vi "save default config.vi"() -> (3 "Data out":T1)   [LabVIEW 2025]
uses:
  safety light settings.ctl
  8253c311-8266-41c7-aa3e-9534f31a7151.vi
  fc13ce0c-d746-4782-a37b-4bbc89a20136.vi
  <vilib>/JDP Science/JSONtext/Variant to JSON Text.vi
  <vilib>/JDP Science/JSONtext/JSON text to Variant.vi
  <vilib>/JDP Science/JSONtext/LVClass Serializer/JSONtext LVClass Serializer.lvclass
panel:
  in  "overwrite file":bool
  in  "default config":T1
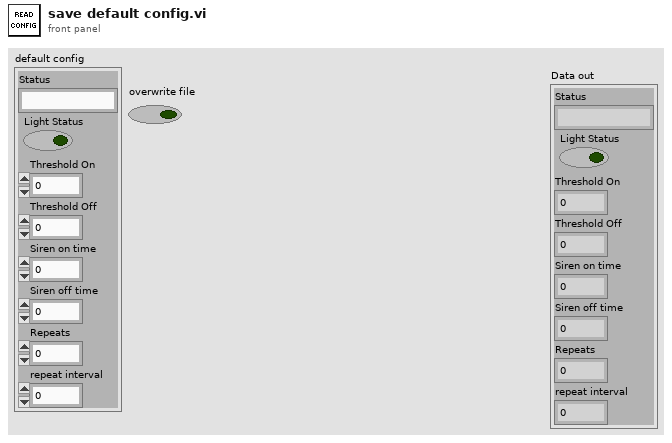
[diagram p1: front panel]
types:
  T1 = typedef "safety light settings.ctl" = cluster{"Status":string, "Light Status":bool, "Threshold On":dbl, "Threshold Off":dbl, "Siren on time":dbl, "Siren off time":dbl, "Repeats":i32, "repeat interval":dbl}
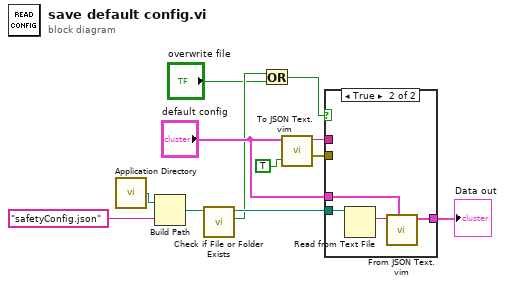
[diagram p0: block diagram]
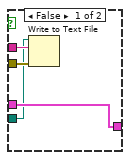
[diagram p2: hidden frame]
diagram:
  n1 = call <vilib>:"Application Directory.vi"() -> ("Application Directory"=w12:path)
  n2 = Build Path(base path=w12, name or relative path="safetyConfig.json" ("JSON string")) -> (appended path=w10:path)
  n3 = call <vilib>:"Check if File or Folder Exists.vi"("path"=w10) -> ("file or folder exists?"=w4:bool, "dup path"=w9:path)  [unwired: 8 in, 1 out]
  n4 = Or(x=w4, y="overwrite file") -> (x .or. y?=w2:bool)
  n5 = call "To JSON Text.vim"("Pretty Print?"=TRUE, "Anything"="default config") -> ("error out"=w6:errorcluster, "<JSON>"=w7:string)  [unwired: 8 in]
  n6 = case shown="True" w2 {
    tunnel: w6 -> [w16 _]
    tunnel: w7 -> [w15 _]
    tunnel: [w14 w17] -> w3
    tunnel: "default config" -> [w14 w18]
    tunnel: w9 -> [w13 w20]
    frame False {
      n7 = Write to Text File(file (use dialog)=w13, text=w15, error in=w16) -> ()  [unwired: 1 in, 3 out]
    }
    frame True {
      n8 = Read from Text File(file (use dialog)=w20) -> (text=w19:string)  [unwired: 3 in, 3 out]
      n9 = call "From JSON Text.vim"("Data Type and Default Value"=w18, "JSON"=w19) -> ("Data out"=w17:T1)  [unwired: 8 in, 1 out]
    }
  }
  "Data out" <- w3
